vi "Temp conversions.vi"() -> ()   [LabVIEW 2014]
panel:
  out "Kelvin":dbl
  out "Farenheit":dbl
  out "Celsius":dbl
  in  "Celsius":dbl
  in  "Farenheit":dbl
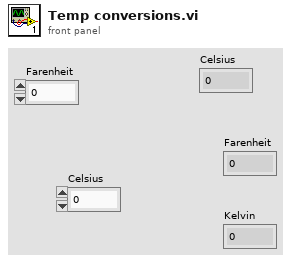
[diagram p1: front panel]
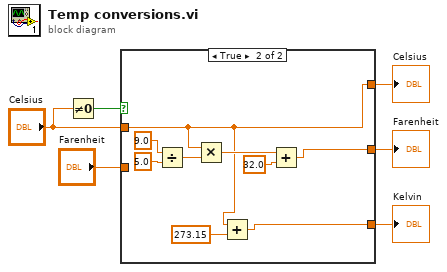
[diagram p0: block diagram]
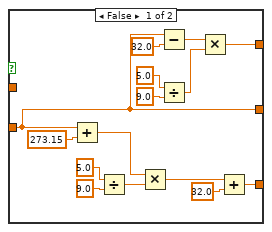
[diagram p2: hidden frame]
diagram:
  n1 = Not Equal To 0?(x="Celsius") -> (x != 0?=w6:bool)
  n2 = case shown="True" w6 {
    tunnel: "Farenheit" -> [w11 _]
    tunnel: "Celsius" -> [_ w24]
    tunnel: [w16 w24] -> w3
    tunnel: [w11 w25] -> w2
    tunnel: [w7 w22] -> w1
    frame False {
      n3 = Add(x=w11, y=273.15) -> (x+y=w12:dbl)
      n4 = Divide(x=5.0, y=9.0) -> (x/y=w13:dbl)
      n5 = Multiply(x=w12, y=w13) -> (x*y=w9:dbl)
      n6 = Subtract(x=w11, y=32.0) -> (x-y=w20:dbl)
      n7 = Divide(x=5.0, y=9.0) -> (x/y=w17:dbl)
      n8 = Multiply(x=w20, y=w17) -> (x*y=w16:dbl)
      n9 = Add(x=w9, y=32.0) -> (x+y=w7:dbl)
    }
    frame True {
      n10 = Divide(x=9.0, y=5.0) -> (x/y=w28:dbl)
      n11 = Multiply(x=w24, y=w28) -> (x*y=w26:dbl)
      n12 = Add(x=w24, y=273.15) -> (x+y=w22:dbl)
      n13 = Add(x=w26, y=32.0) -> (x+y=w25:dbl)
    }
  }
  "Kelvin" <- w1
  "Farenheit" <- w2
  "Celsius" <- w3
